vi "Start Core.vi"(8 "error in (no error)":errorcluster, 11 "VolatusCore in":refnum<class "VolatusCore.lvclass">) -> (0 "error out":errorcluster, 3 "VolatusCore out":refnum<class "VolatusCore.lvclass">)   [LabVIEW 2020, in "Volatus.lvlib" / "VolatusCore.lvclass"]
uses:
  VolatusCore.lvclass
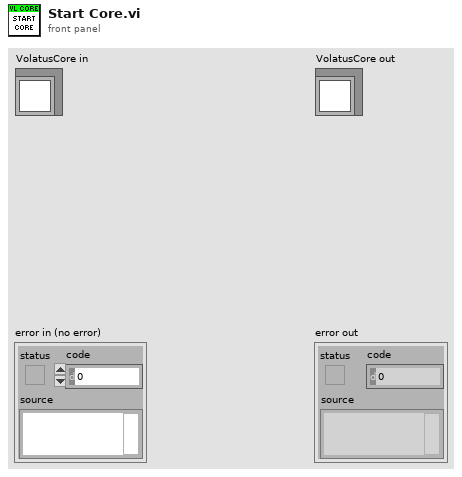
[diagram p1: front panel]
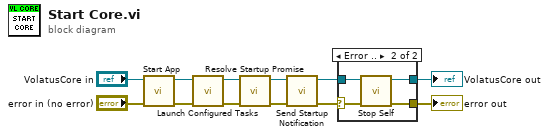
[diagram p0: block diagram]
diagram:
  n1 = call "Start App.vi"("error in (no error)"="error in (no error)", "VolatusCore in"="VolatusCore in") -> ("error out"=w12:errorcluster, "VolatusCore out"=w5:refnum<class "VolatusCore.lvclass">)  [unwired: 8 in]
  n2 = call "Launch Configured Tasks.vi"("error in (no error)"=w12, "VolatusCore in"=w5) -> ("error out"=w6:errorcluster, "VolatusCore out"=w4:refnum<class "VolatusCore.lvclass">)  [unwired: 8 in]
  n3 = call "Resolve Startup Promise.vi"("error in (no error)"=w6, "VolatusCore in"=w4) -> ("error out"=w11:errorcluster, "VolatusCore out"=w10:refnum<class "VolatusCore.lvclass">)  [unwired: 8 in]
  n4 = call "Send Startup Notification.vi"("error in (no error)"=w11, "VolatusCore in"=w10) -> ("error out"=w7:errorcluster, "VolatusCore out"=w2:refnum<class "VolatusCore.lvclass">)  [unwired: 8 in]
  n5 = case shown="Error .." w7 {
    selector: w7 -> [w13 w18]
    tunnel: [w13 w17] -> w3
    tunnel: w2 -> [w14 w16]
    tunnel: [w14 w15] -> w1
    frame No Error {
    }
    frame Error {
      n6 = call "Stop Self.vi"("error in (no error)"=w18, "VolatusCore in"=w16) -> ("error out"=w17:errorcluster, "VolatusCore out"=w15:refnum<class "VolatusCore.lvclass">)  [unwired: 8 in]
    }
  }
  "error out" <- w3
  "VolatusCore out" <- w1
